vi "create error request.vi"(7 "incoming request":T1, 9 "lv error description":string, 10 "reason":string, 11 "code":string) -> (3 "element":T1)   [LabVIEW 2016, in "Basic HTTPS server.lvclass"]
uses:
  Basic HTTPS server.lvclass
  http request.ctl
  http method.ctl
  HTTP headers/http header data.ctl
  HTTP headers/http headers.lvlib
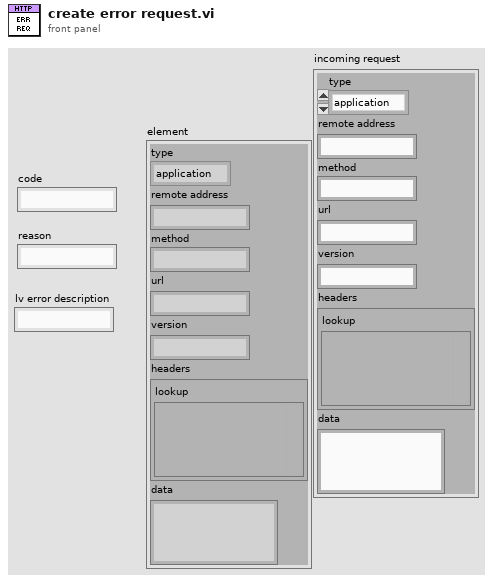
[diagram p1: front panel]
types:
  T1 = typedef "Basic HTTPS server.lvclass/http request.ctl" = cluster{"type":T2, "remote address":string, "method":string, "url":string, "version":string, "headers":T3, "data":string}
  T2 = typedef "Basic HTTPS server.lvclass/http method.ctl" = enum16{"application", "error", "upgrade"}
  T3 = typedef "http headers.lvlib/http header data.ctl" = cluster{"lookup":variant}
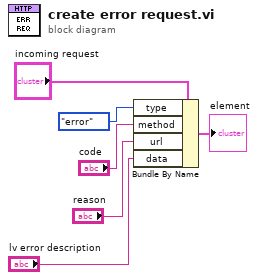
[diagram p0: block diagram]
diagram:
  n1 = Bundle By Name(cluster="incoming request", "type"=http_method."error", "method"="code", "url"="reason", "data"="lv error description") -> (→"element":T1)
